vi "DashboardGetSafetyStatus.vi"(8 "Dashboard":refnum<k24>, 11 "error in":errorcluster) -> (0 "Response":cluster{"Message":string, "Succeed":bool}, 1 "status":u8(ring)=1 items=["Normal"=1, "Reduced"=2, "ProtectiveStop"=3, "Recovery"=4, "SafeguardStop"=5, "SystemEmergencyStop"=6, "RobotEmergencyStop"=7, "Violation"=8, "Fault"=9, "AutomaticModeSafeguardStop"=10, "SystemThreePositionEnablingStop"=11], 3 "error out":errorcluster)   [LabVIEW 2013, in "UnderAutomation.UniversalRobots.lvlib"]
uses:
  UnderAutomation.UniversalRobots.lvlib
  C:/Users/fg/Documents/UniversalRobots.vi/LabVIEW_2024/UnderAutomation.UniversalRobots/lib/UnderAutomation.UniversalRobots.dll
  LabVIEW_2024/UnderAutomation.UniversalRobots/lib/UnderAutomation.UniversalRobots.dll
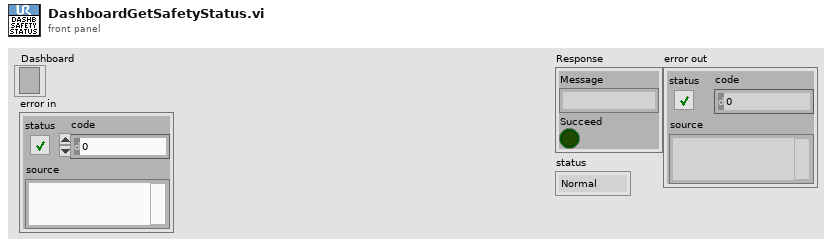
[diagram p1: front panel]
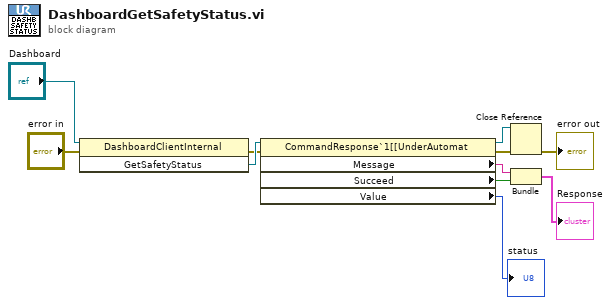
[diagram p0: block diagram]
diagram:
  n1 = invoke class="DashboardClientInternal" method="GetSafetyStatus"(reference="Dashboard", error in="error in") -> (error out=w5:errorcluster, "GetSafetyStatus"=w10:refnum<k24>)  [unwired: 1 in, 1 out]
  n2 = property class="CommandResponse`1[[UnderAutomat"(reference=w10, error in=w5) -> (reference out=w1:refnum<k24>, error out=w3:errorcluster, "Message"=w9:string, "Succeed"=w8:bool, "Value"=→"status":u8)
  n3 = Close Reference(reference=w1, error in (no error)=w3) -> (error out=→"error out":errorcluster)
  n4 = Bundle("Message"=w9, "Succeed"=w8) -> (→"Response":cluster{"Message":string, "Succeed":bool})  [unwired: 1 in]
